vi "TestVirtual5.vi"(0 "reference in":refnum<class "G#SubSubClass1.lvclass">, 5 "error in (no error)":errorcluster) -> (14 "reference out":refnum<class "G#SubSubClass1.lvclass">, 15 "MethodName":string[](array[string]), 19 "error out":errorcluster)   [LabVIEW 2010, in "G#SubSubClass1.lvclass"]
uses:
  G#SubSubClass1.lvclass
  G#SubClass1_class/G#SubClass1.lvclass
  G#BaseClass1_class/G#BaseClass1.lvclass
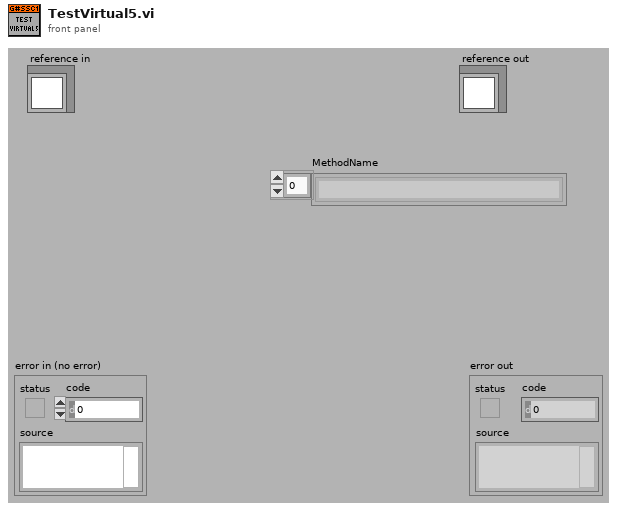
[diagram p1: front panel]
types:
  T1 = typedef "G#SubSubClass1.lvclass/ObjectAttributes.ctl" = cluster{"Numeric":dbl, "G#BaseClass1.lvclass":refnum<class "G#BaseClass1.lvclass">}
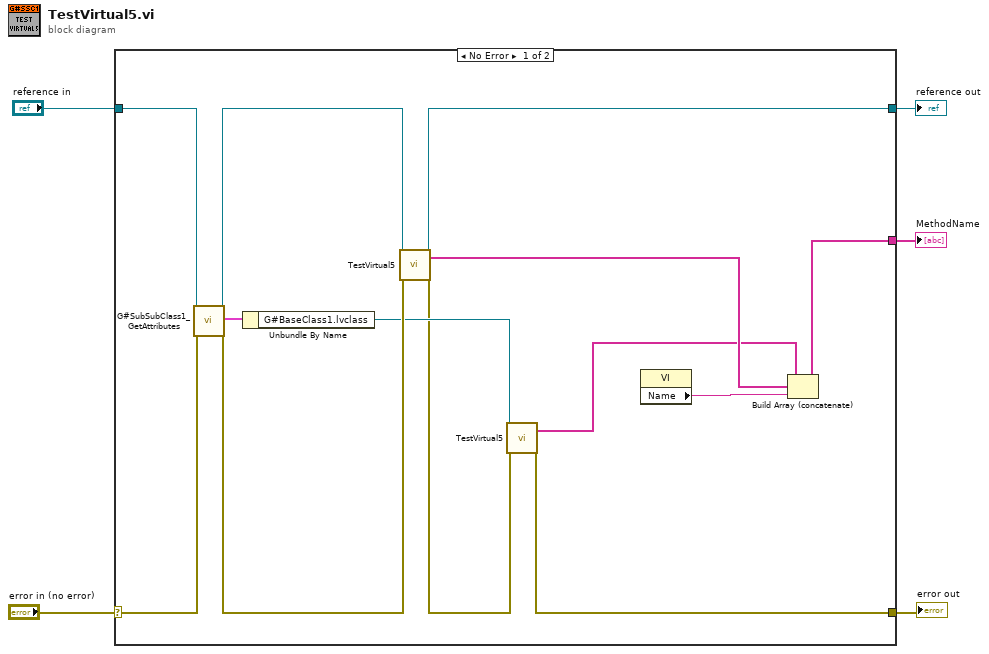
[diagram p0: block diagram]
diagram:
  n1 = case shown="No Error" "error in (no error)" {
    selector: "error in (no error)" -> [w13 w20]
    tunnel: [w8 w20] -> w4
    tunnel: [w18 w19] -> w2
    tunnel: "reference in" -> [w15 w19]
    tunnel: [w16 _] -> w1
    frame No Error {
      n2 = call "G#SubSubClass1_GetAttributes.vi"("reference in"=w15, "error in (no error)"=w13) -> ("reference out"=w14:refnum<class "G#SubSubClass1.lvclass">, "attributes"=w11:T1, "error out"=w12:errorcluster)  [unwired: 14 in, 1 out]
      n3 = Unbundle By Name(w11) -> ("G#BaseClass1.lvclass"=w10:refnum<class "G#BaseClass1.lvclass">)
      n4 = call-parent "TestVirtual5.vi"("reference in"=w14, "error in (no error)"=w12) -> ("reference out"=w18:refnum<class "G#SubSubClass1.lvclass">, "MethodName"=w7:string[], "error out"=w9:errorcluster)  [unwired: 15 in]
      n5 = call-dynamic "TestVirtual5.vi"("reference in"=w10, "error in (no error)"=w9) -> ("MethodName"=w6:string[], "error out"=w8:errorcluster)  [unwired: 15 in, 1 out]
      n6 = property class="VI"() -> ("Name"=w17:string)  [unwired: 2 in, 2 out]
      n7 = Build Array (concatenate)(w6, w7, w17) -> (w16:string[])
    }
    frame Error {
    }
  }
  "error out" <- w4
  "reference out" <- w2
  "MethodName" <- w1
